vi "Set SndPB - Parameters.vi"(0 "reference in":refnum<class "GSwFormDSP.lvclass">, 5 "error in (no error)":errorcluster, 7 "Sound Playback":T1={"Timer start (ms)"=0, "task ID"=0, "Cursor Init Location (s)"=1.0, "SC Volume"=100.0} {"SC Volume" scale=0.0..100.0; "task ID" format="%.0x"}) -> (14 "reference out":refnum<class "GSwFormDSP.lvclass">, 19 "error out":errorcluster)   [LabVIEW 2020, in "GSwFormDSP.lvclass"]
uses:
  GSwFormDSP.lvclass
  functions/Sound Playback.ctl
  <vilib>/sound2/lvsound2.llb/Sound Output Task ID.ctl
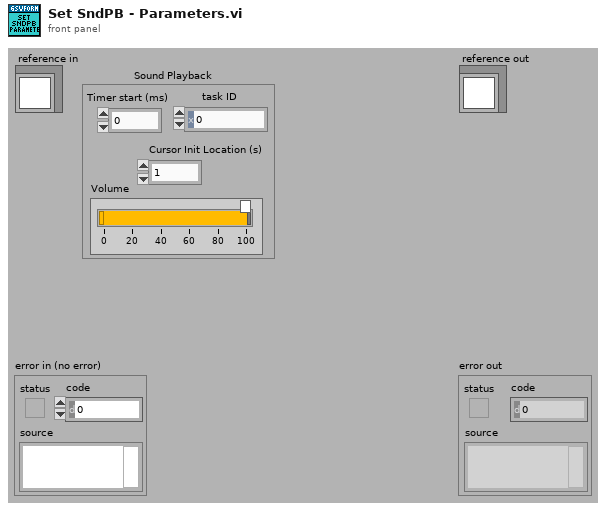
[diagram p1: front panel]
types:
  T1 = typedef "GSwFormDSP.lvclass/Sound Playback.ctl" = cluster{"Timer start (ms)":u32, "task ID":T2, "Cursor Init Location (s)":dbl, "SC Volume":dbl}
  T2 = typedef "Sound Output Task ID.ctl" = u32
  T3 = typedef "GSwFormDSP.lvclass/ObjectAttributesRef.ctl" = refnum<data-value>
  T4 = typedef "GSwFormDSP.lvclass/ObjectAttributes.ctl" = cluster{"Wform Ref":refnum<data-value>, "Nb Signals":i32, "Spectral Function Parameters":T5, "FFT":waveform(cdb)[], "Nb FFT":i32, "Nb Averages":i32[], "Reference Indexes":i32[], "Response Indexes":i32[], "Coherence":waveform(dbl)[], "TDF Parameters":T7, "DAQ":cluster{"Duration (sec)":dbl, "Buffer Size (Samples)":i32, "Offset (Samples)":i32}, "Filter Impulse Response (TDF)":waveform(dbl), "Sound Playback":T1}
  T5 = typedef "GSwFormDSP.lvclass/Spectral Parameters.ctl" = cluster{"Frequency resolution (Hz)":dbl, "Overlap":dbl, "Window":T6}
  T6 = typedef "NI_AALPro.lvlib/windowTd.ctl" = u32
  T7 = typedef "GSwFormDSP.lvclass/TDF Parameters.ctl" = cluster{"Filter":enum32{"Lowpass", "Highpass", "Bandpass", "Bandstop"}, "Type:":enum16{"Butterworth", "Chebyshev", "Inv Chebyshev", "Elliptic", "Bessel"}, "LP cutoff freq":dbl, "HP cutoff freq":dbl, "Order":i32, "passband ripple (dB)":dbl, "stopband attenuation (dB)":dbl, "Phaseless Filter":bool, "Include Fade IN and OUT":bool}
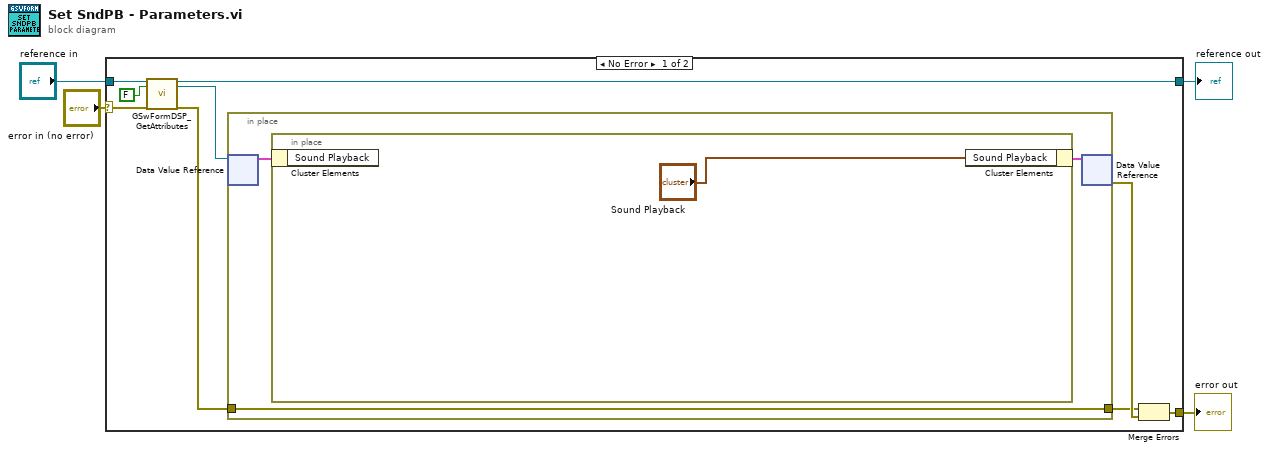
[diagram p0: block diagram]
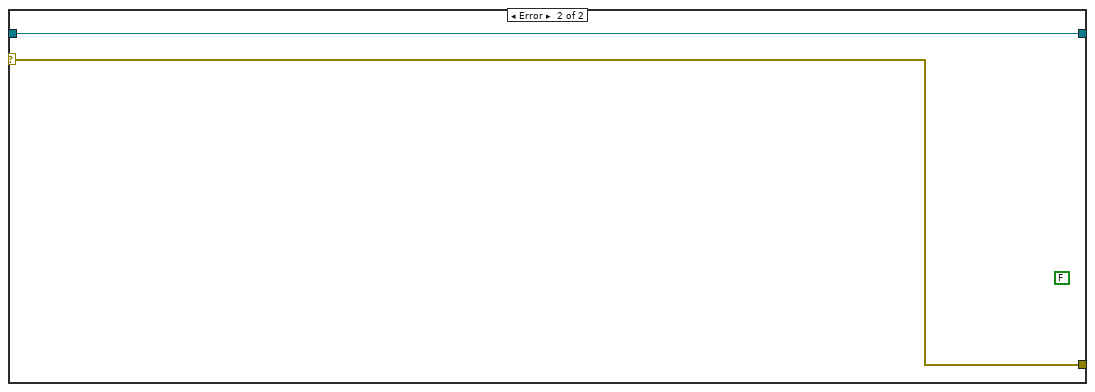
[diagram p2: hidden frame]
diagram:
  n1 = case shown="No Error" "error in (no error)" {
    selector: "error in (no error)" -> [w6 w19]
    tunnel: [w13 w19] -> w3
    tunnel: [w8 w18] -> w1
    tunnel: "reference in" -> [w5 w18]
    frame No Error {
      n2 = call "GSwFormDSP_GetAttributes.vi"("reference in"=w5, "return data? (T)"=FALSE, "error in (no error)"=w6) -> ("reference out"=w8:refnum<class "GSwFormDSP.lvclass">, "attributes ref"=w7:T3, "error out"=w9:errorcluster)  [unwired: 13 in, 1 out]
      n3 = in-place {
        in-place-border: w9 -> [w14]
        in-place-border: [w14] -> w11
        n4 = in-place-dvr #1(w7) -> (w15:T4)  [unwired: 1 out]
        n5 = in-place {
          n6 = in-place-cluster #2(w15) -> ()  [unwired: 1 out]
          n7 = in-place-cluster #2("Sound Playback"="Sound Playback") -> (w16:T4)
        }
        n8 = in-place-dvr #1(w16) -> (w12:errorcluster)  [unwired: 1 out]
      }
      n9 = Merge Errors(w11, w12) -> (w13:errorcluster)
    }
    frame Error {
      (unwired) FALSE
    }
  }
  "error out" <- w3
  "reference out" <- w1
